vi "EnableDisableLogging.vi"(7 "LabVIEW Web Service Request":refnum<class "Web Request.lvclass">) -> ()   [LabVIEW 2018]
uses:
  <vilib>/wsapi/Web Request.lvclass
  CAEN globals.vi
panel:
  in  "error in (no error)":errorcluster
  # "Use the Web Service Request input terminal to call the VIs on the Web Services palette. Do not remove it from the connector pane unless you don't need access to the palette."
  # "Each additional control wired to the connector pane will be available as an input in the URL. To include an indicator in terminal-mode output (the default setting), it must also be wired to the connector pane."
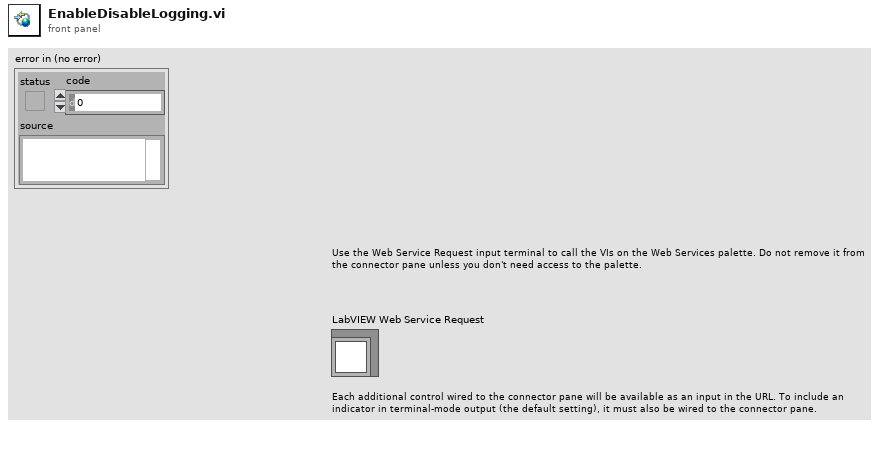
[diagram p1: front panel]
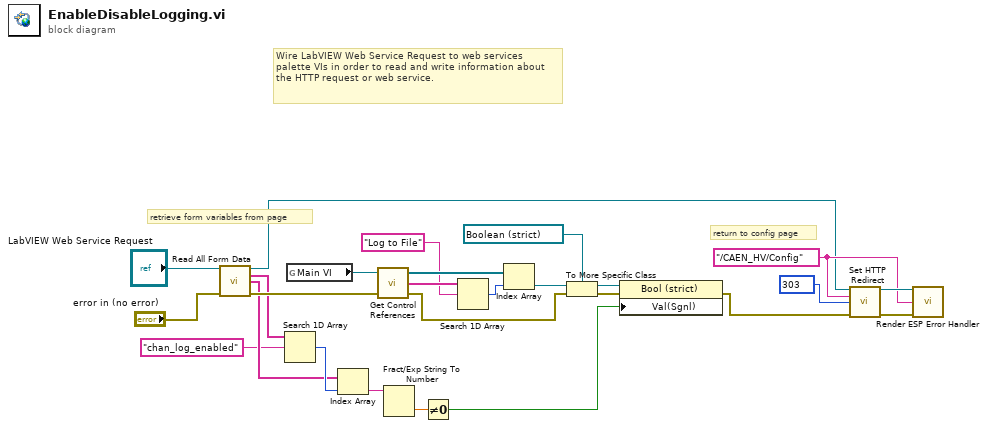
[diagram p0: block diagram]
diagram:
  w16 = 303 items=["100"=100, "101"=101, "200"=200, "201"=201, "202"=202, "203"=203, "204"=204, "205"=205, "206"=206, "300"=300, "301"=301, "302"=302, "303"=303, "304"=304, "305"=305, "306"=306, "307"=307, "400"=400, "401"=401, "402"=402, "403"=403, "404"=404, "405"=405, "406"=406, "407"=407, "408"=408, "409"=409, "410"=410, "411"=411, "412"=412, "413"=413, "414"=414, "415"=415, "416"=416, "417"=417, "500"=500, "501"=501, "502"=502, "503"=503, "504"=504, "505"=505] ("response code (307)")
  w12 = "/CAEN_HV/Config" ("redirect URL")
  # "retrieve form variables from page"
  # "return to config page"
  # "Wire LabVIEW Web Service Request to web services palette VIs in order to read and write information about the HTTP request or web service."
  n1 = call <vilib>:"Read All Form Data.vi"("LabVIEW Web Service Request"="LabVIEW Web Service Request", "error in (no error)"="error in (no error)") -> ("LabVIEW Web Service Request out"=w8:refnum<class "Web Request.lvclass">, "Key"=w7:string[], "Value"=w5:string[], "error out"=w9:errorcluster)  [unwired: 9 in, 1 out]
  n2 = Search 1D Array(1D array=w7, element="chan_log_enabled") -> (index of element=w6:i32)  [unwired: 1 in]
  n3 = global read "CAEN globals.vi" "Main VI"() -> (w26:refnum<vi>)
  n4 = Index Array(array=w5, index=w6) -> (element=w4:string)
  n5 = call "Get Control References.vi"("error in"=w9, "This vi"=w26) -> ("error out"=w17:errorcluster, "Control Names"=w25:string[], "Controls[]"=w24:refnum<vi>[])  [unwired: 1 in]
  n6 = Fract/Exp String To Number(string=w4) -> (number=w3:dbl)  [unwired: 3 in, 1 out]
  n7 = Not Equal To 0?(x=w3) -> (x != 0?=w2:bool)
  n8 = Search 1D Array(1D array=w25, element="Log to File" ("Label.Text")) -> (index of element=w20:i32)  [unwired: 1 in]
  n9 = Index Array(array=w24, index=w20) -> (element=w18:refnum<vi>)
  n10 = To More Specific Class(target class=refnum<vi> refnum ("replace all? (F)"), reference=w18, error in=w17) -> (specific class reference=w22:refnum<vi>, error out=w23:errorcluster)
  n11 = property class="Bool (strict)"(reference=w22, error in=w23, "Val(Sgnl)"=w2) -> (error out=w13:errorcluster)  [unwired: 1 out]
  n12 = call <vilib>:"Set HTTP Redirect.vi"("LabVIEW Web Service Request"=w8, "redirect URL"=w12, "response code (307)"=w16, "error in (no error)"=w13) -> ("LabVIEW Web Service Request out"=w14:refnum<class "Web Request.lvclass">, "error out"=w15:errorcluster)  [unwired: 10 in]
  n13 = call "Render ESP Error Handler.vi"("LabVIEW Web Service Request"=w14, "Link"=w12, "error in (no error)"=w15) -> ()  [unwired: 11 in, 2 out]
